vi "Main.vi"   [LabVIEW 2011]
uses:
  <vilib>/measure/NI_MABase.lvlib
panel:
  # "This is MainVI"
types:
  T1 = cluster{"signal type":enum16{"Sine Wave", "Triangle Wave", "Square Wave", "Sawtooth Wave"}, "frequency":dbl, "amplitude":dbl, "signal out":waveform(dbl), "WavefromRefnum":refnum<vi>}
  T2 = enum16{"Sine Wave", "Triangle Wave", "Square Wave", "Sawtooth Wave"}
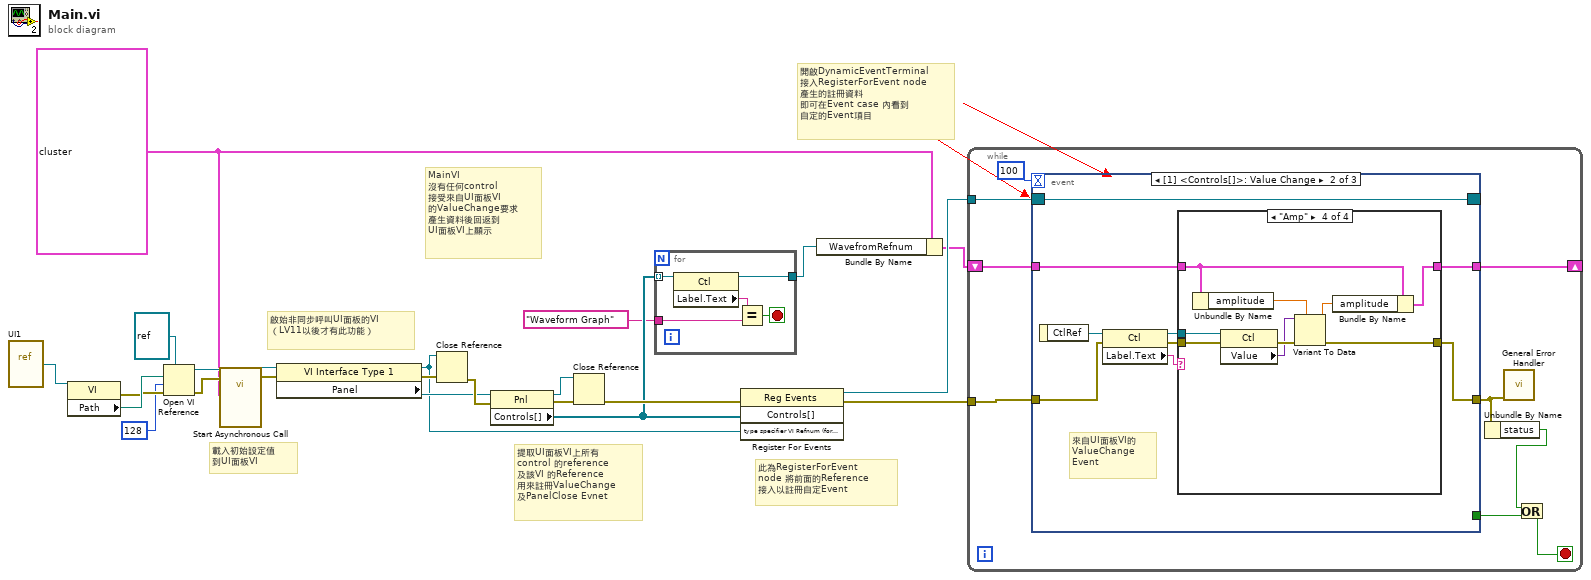
[diagram p0: block diagram]
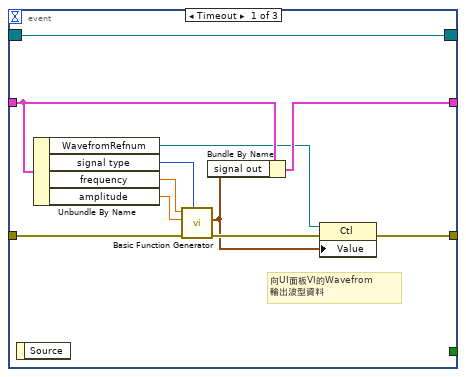
[diagram p2: hidden frame]
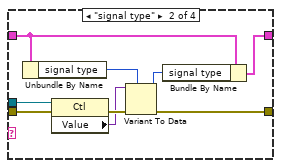
[diagram p4: hidden frame]
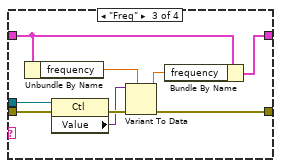
[diagram p5: hidden frame]
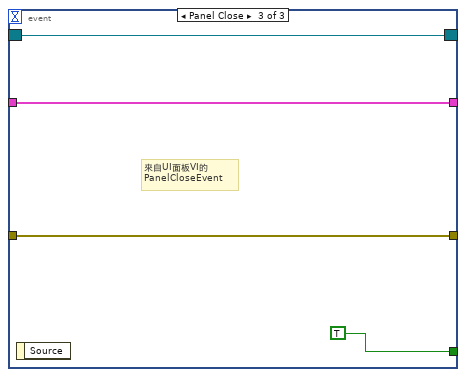
[diagram p6: hidden frame]
diagram:
  w1 = T1 {"signal type"=enum."Sine Wave", "frequency"=3.1, "amplitude"=1.414, "signal out"={"t0"=timestamp(0 s since 1904-01-01), "dt"=1.0, "Y"=[]}, "WavefromRefnum"=refnum}
  # "載入初始設定值\n到UI面板VI"
  # "MainVI\n沒有任何control\n接受來自UI面板VI\n的ValueChange要求\n產生資料後回返到\nUI面板VI上顯示"
  # "開啟DynamicEventTerminal\n接入RegisterForEvent node\n產生的註冊資料\n即可在Event case 內看到\n自定的Event項目"
  # "此為RegisterForEvent\nnode 將前面的Reference\n接入以註冊自定Event"
  # "提取UI面板VI上所有\ncontrol 的reference\n及該VI 的Reference\n用來註冊ValueChange\n及PanelClose Evnet"
  # "啟始非同步呼叫UI面板的VI\n（LV11以後才有此功能）"
  n1 = vi-ref "UI1.vi"() -> (w23:refnum<vi>)
  n2 = property class="VI"(reference=w23) -> (error out=w21:errorcluster, "Path"=w22:path)  [unwired: 1 in, 1 out]
  n3 = Open VI Reference(type specifier VI Refnum (for type only)=refnum<vi> refnum, vi path=w22, options=128, error in (no error)=w21) -> (vi reference=w20:refnum<vi>, error out=w18:errorcluster)  [unwired: 2 in]
  n4 = call-by-ref "Start Asynchronous Call"(reference=w20, error in=w18, "Cluster"=w1) -> (reference out=w17:refnum<vi>, error out=w16:errorcluster)  [unwired: 9 in]
  n5 = property class="VI Interface Type 1"(reference=w17, error in=w16) -> (reference out=w9:refnum<vi>, error out=w15:errorcluster, "Panel"=w13:refnum<vi>)
  n6 = Close Reference(reference=w9, error in (no error)=w15) -> (error out=w14:errorcluster)
  n7 = property class="Pnl"(reference=w13, error in=w14) -> (reference out=w7:refnum<vi>, error out=w12:errorcluster, "Controls[]"=w6:refnum<vi>[])
  n8 = Close Reference(reference=w7, error in (no error)=w12) -> (error out=w8:errorcluster)
  n9 = for {
    tunnel: w6 -> [w28] mode=indexing
    tunnel: "Waveform Graph" ("Label.Text") -> [w26]
    tunnel: [w24] -> w4
    stop <- w25 stop-if-true
    n10 = property class="Ctl"(reference=w28) -> (reference out=w24:refnum<vi>, "Label.Text"=w27:string)  [unwired: 1 in, 1 out]
    n11 = Equal?(x=w27, y=w26) -> (x = y?=w25:bool)
  }
  n12 = register-events(error in=w8, w6, w9) -> (reference out=w11:refnum<event-registration>, error out=w10:errorcluster)  [unwired: 1 in]
  n13 = Bundle By Name(cluster=w1, "WavefromRefnum"=w4) -> (w3:T1)
  n14 = while {
    tunnel: w11 -> [w37]
    tunnel: w10 -> [w36]
    shift-right: [w32] -> _
    shift-left: w3 -> [w33]
    stop <- w30 stop-if-true
    n15 = event shown="[1] <Controls[]>: Value Change" {
      selector: w37 -> [w48 w57 w89]
      dyn-events: [w48 w57 w89] -> _
      timeout: 100 -> [_ _ _]
      tunnel: w36 -> [w44 w55 w87]
      tunnel: [_ _ TRUE ("Discard?")] -> w35
      tunnel: w33 -> [w42 w53 w88]
      tunnel: [w40 w49 w87] -> w31
      tunnel: [w41 w50 w88] -> w32
      event Timeout {
        # "向UI面板VI的Wavefrom\n輸出波型資料"
        n16 = event-data() -> ()  [unwired: 1 in, 1 out]
        n17 = Unbundle By Name(w42) -> ("WavefromRefnum"=w39:refnum<vi>, "signal type"=w47:T2, "frequency"=w46:dbl, "amplitude"=w45:dbl)
        n18 = call <vilib>:"Basic Function Generator.vi"("signal type"=w47, "error in (no error)"=w44, "amplitude"=w45, "frequency"=w46) -> ("error out"=w43:errorcluster, "signal out"=w38:waveform(dbl))  [unwired: 5 in, 1 out]
        n19 = Bundle By Name(cluster=w42, "signal out"=w38) -> (w41:T1)
        n20 = property class="Ctl"(reference=w39, error in=w43, "Value"=w38) -> (error out=w40:errorcluster)  [unwired: 1 out]
      }
      event Value Change {
        # "來自UI面板VI的\nValueChange \nEvent"
        n21 = event-data() -> ("CtlRef"=w56:refnum<vi>)  [unwired: 1 in]
        n22 = property class="Ctl"(reference=w56, error in=w55) -> (reference out=w52:refnum<vi>, error out=w51:errorcluster, "Label.Text"=w54:string)
        n23 = case shown="\"Amp\"" w54 {
          tunnel: w53 -> [w59 w63 w72 w81]
          tunnel: w52 -> [_ w68 w77 w86]
          tunnel: w51 -> [w58 w67 w76 w85]
          tunnel: [w59 w61 w70 w79] -> w50
          tunnel: [w58 w60 w69 w78] -> w49
          frame Default {
          }
          frame "signal type" {
            n24 = Unbundle By Name(w63) -> ("signal type"=w64:T2)
            n25 = property class="Ctl"(reference=w68, error in=w67) -> (error out=w66:errorcluster, "Value"=w65:variant)  [unwired: 1 out]
            n26 = Variant To Data(error in=w66, type=w64, Variant=w65) -> (data=w62:T2, error out=w60:errorcluster)
            n27 = Bundle By Name(cluster=w63, "signal type"=w62) -> (w61:T1)
          }
          frame "Freq" {
            n28 = Unbundle By Name(w72) -> ("frequency"=w73:dbl)
            n29 = property class="Ctl"(reference=w77, error in=w76) -> (error out=w75:errorcluster, "Value"=w74:variant)  [unwired: 1 out]
            n30 = Variant To Data(error in=w75, type=w73, Variant=w74) -> (data=w71:dbl, error out=w69:errorcluster)
            n31 = Bundle By Name(cluster=w72, "frequency"=w71) -> (w70:T1)
          }
          frame "Amp" {
            n32 = Unbundle By Name(w81) -> ("amplitude"=w82:dbl)
            n33 = property class="Ctl"(reference=w86, error in=w85) -> (error out=w84:errorcluster, "Value"=w83:variant)  [unwired: 1 out]
            n34 = Variant To Data(error in=w84, type=w82, Variant=w83) -> (data=w80:dbl, error out=w78:errorcluster)
            n35 = Bundle By Name(cluster=w81, "amplitude"=w80) -> (w79:T1)
          }
        }
      }
      event Panel Close {
        # "來自UI面板VI的\nPanelCloseEvent"
        n36 = event-data() -> ()  [unwired: 1 in, 1 out]
      }
    }
    n37 = Unbundle By Name(w31) -> ("status"=w29:bool)
    n38 = call <vilib>:"General Error Handler.vi"("error in (no error)"=w31) -> ()  [unwired: 10 in, 5 out]
    n39 = Or(x=w29, y=w35) -> (x .or. y?=w30:bool)
  }
